vi "AlazarDSPGetNextBufferU8.vi"(4 "error in (no error)":errorcluster, 5 "timeout_ms":u32, 6 "Buffer":u8[](array[numeric]), 7 "Handle":u64) -> (0 "error out":errorcluster, 1 "Return Code":u32, 2 "Buffer":u8[](array[numeric]), 3 "Handle":u64)   [LabVIEW 2009]
doc: "This function returns when the board has received sufficient trigger events to fill the buffer, or the timeout interval has elapsed. To use this function, AlazarBeforeAsyncRead must be called with the ADMA_ALLOC_BUFFERS flag."
uses:
  ATSApi.dll
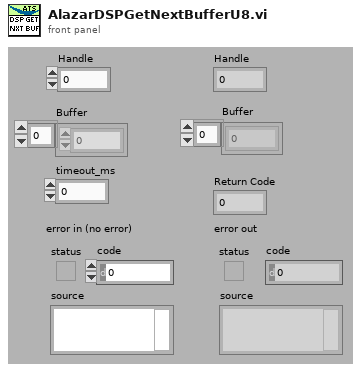
[diagram p1: front panel]
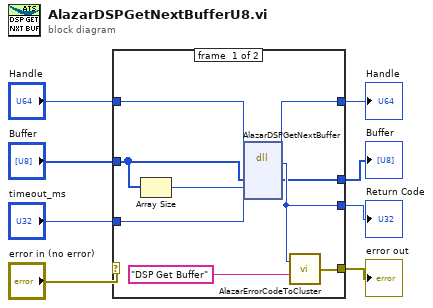
[diagram p0: block diagram]
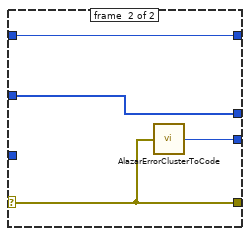
[diagram p2: hidden frame]
diagram:
  n1 = case shown="No Error" "error in (no error)" {
    selector: "error in (no error)" -> [_ w21]
    tunnel: [w14 w21] -> w7
    tunnel: [w16 w20] -> w6
    tunnel: "Handle" -> [w17 w19]
    tunnel: [w13 w19] -> w4
    tunnel: "Buffer" -> [w10 w18]
    tunnel: "timeout_ms" -> [w11 _]
    tunnel: [w12 w18] -> w1
    frame #0 {
      n2 = Array Size(array=w10) -> (size(s)=w9:i32)
      n3 = dll-call lib="ATSApi.dll" fn="AlazarDSPGetNextBuffer"("handle"=w17, "buffer"=w10, "bytesToCopy"=w9, "timeout_ms"=w11) -> ("return type"=w16:u32, "handle"=w13:u64, "buffer"=w12:u8[])  [unwired: 5 in, 2 out]
      n4 = call "AlazarErrorCodeToCluster.vi"("Message"="DSP Get Buffer", "Error Code"=w16) -> ("error out"=w14:errorcluster)
    }
    frame #1 {
      n5 = call "AlazarErrorClusterToCode.vi"("error in (no error)"=w21) -> ("Error Code"=w20:u32)
    }
  }
  "Handle" <- w4
  "error out" <- w7
  "Return Code" <- w6
  "Buffer" <- w1
